vi "close.vi"(8 "error in":errorcluster, 10 "data":variant) -> (0 "error out":errorcluster)   [LabVIEW 2018, in "Sensor Interface.lvlib"]
doc: "This VI enqueues the named action"
uses:
  Sensor Interface.lvlib
  Private Controls/Module Data Cluster.ctl
  Private Controls/Module Action.ctl
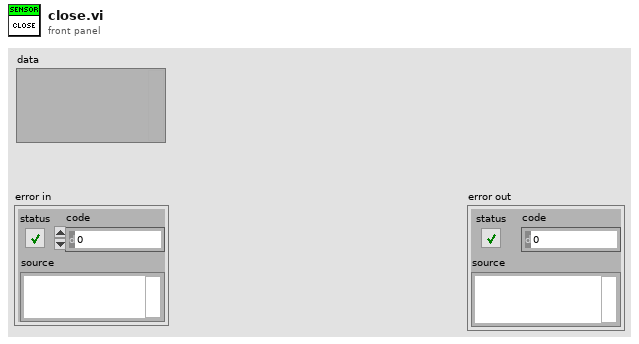
[diagram p1: front panel]
types:
  T1 = typedef "Sensor Interface.lvlib/Module Data Cluster.ctl" = cluster{"Variant":variant, "action":T2}
  T2 = typedef "Sensor Interface.lvlib/Module Action.ctl" = enum16{"error", "exit", "init", "Start Sim", "Update Position"}
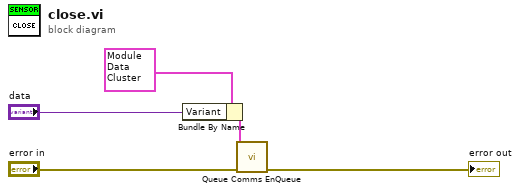
[diagram p0: block diagram]
diagram:
  n1 = Bundle By Name(cluster=T1 {"Variant"=variant, "action"=enum."exit"} ("Module Data Cluster"), "Variant"="data") -> (w4:T1)
  n2 = call "Queue Comms EnQueue.vi"("error in"="error in", "Module Data Cluster"=w4) -> ("error out"=→"error out":errorcluster)  [unwired: 9 in]
